vi "Get UUID.vi"(8 "error in (no error)":errorcluster, 11 "input in":refnum<class "input.lvclass">) -> (0 "error out":errorcluster, 2 "UUID":string, 3 "input out":refnum<class "input.lvclass">)   [LabVIEW 2015, in "input.lvclass"]
uses:
  input.lvclass
  input.lvclass/input.ctl
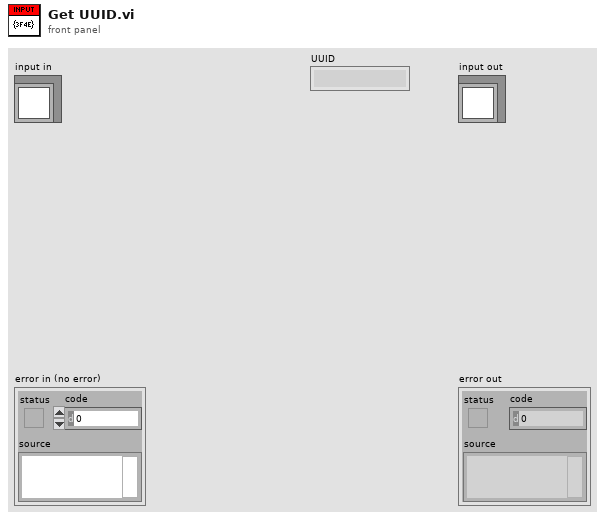
[diagram p1: front panel]
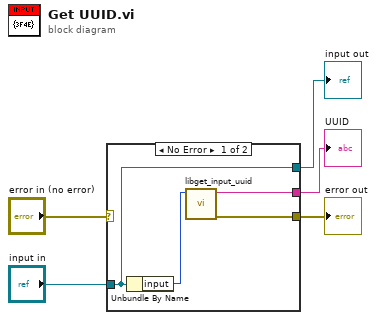
[diagram p0: block diagram]
diagram:
  n1 = case shown="No Error" "error in (no error)" {
    selector: "error in (no error)" -> [_ w11]
    tunnel: [w7 w11] -> w4
    tunnel: [w9 w10] -> w2
    tunnel: "input in" -> [w9 w10]
    tunnel: [w6 _] -> w1
    frame No Error {
      n2 = Unbundle By Name(w9) -> ("input"=w8:i32)
      n3 = call "libget_input_uuid.vi"("input"=w8) -> ("error out"=w7:errorcluster, "UUID"=w6:string)  [unwired: 9 in]
    }
    frame Error {
    }
  }
  "error out" <- w4
  "input out" <- w2
  "UUID" <- w1
